vi "Image_Pro_controls_from_string.vi"(11 "Setup String":string) -> (0 "ROI to crop (pixels)":T2={"Xmax"=2147483647, "Ymax"=2147483647, "Xmin"=0, "Ymin"=0}, 1 "Txy range (pixels)":T3={"Tx max (pix)"=2147483647, "Tx min (pix)"=-2147483648, "Ty max (pix)"=2147483647, "Ty min (pix)"=-2147483648}, 2 "Theta range (deg)":T5={"theta max (deg)"=180.0, "theta min (deg)"=-180.0} {"theta min (deg)" min=-360.0 max=360.0; "theta max (deg)" min=-360.0 max=360.0}, 3 "Controls":T4={"Auto ROI (for rot.)"=FALSE, "Apply scaling"=FALSE, "Apply rotation"=TRUE, "Apply Tx"=TRUE, "Apply Ty"=TRUE, "Keep proc. img"=FALSE}, 4 "Camera":string, 5 "Quality":u32=750 max=1000, 7 "Resolution":T1 items=["Low", "Med.", "High", "Max."])   [LabVIEW 2015]
uses:
  Typedefs/Theta range.ctl
  Typedefs/Top level controls.ctl
  Typedefs/Txy range.ctl
  Typedefs/ROI bounds.ctl
  Camera Server/Camera enum/Camera resolution.ctl
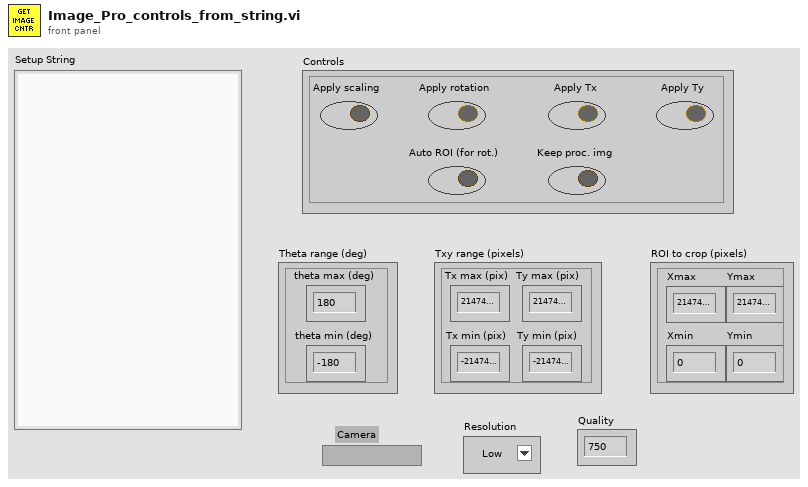
[diagram p1: front panel]
types:
  T1 = typedef "Camera resolution.ctl" = u8
  T2 = typedef "ROI bounds.ctl" = cluster{"Xmax":i32, "Ymax":i32, "Xmin":i32, "Ymin":i32}
  T3 = typedef "Txy range.ctl" = cluster{"Tx max (pix)":i32, "Tx min (pix)":i32, "Ty max (pix)":i32, "Ty min (pix)":i32}
  T4 = typedef "Top level controls.ctl" = cluster{"Auto ROI (for rot.)":bool, "Apply scaling":bool, "Apply rotation":bool, "Apply Tx":bool, "Apply Ty":bool, "Keep proc. img":bool}
  T5 = typedef "Theta range.ctl" = cluster{"theta max (deg)":dbl, "theta min (deg)":dbl}
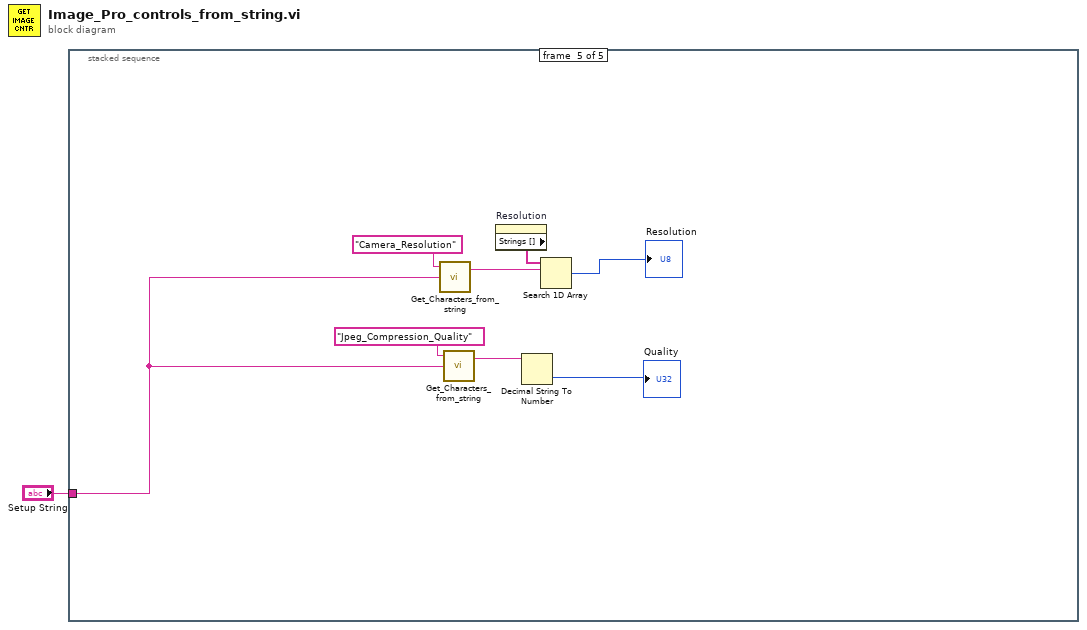
[diagram p0: block diagram]
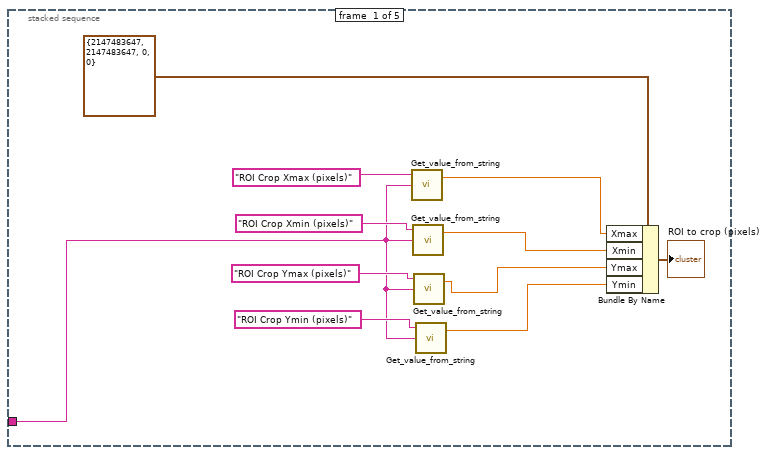
[diagram p2: hidden frame]
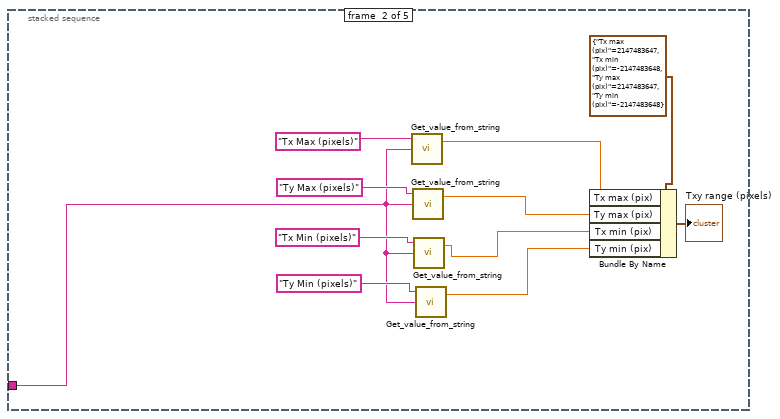
[diagram p3: hidden frame]
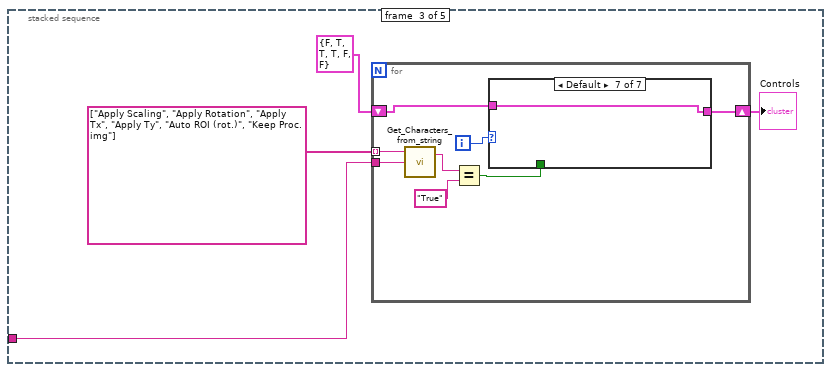
[diagram p4: hidden frame]
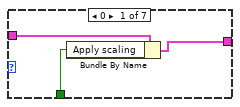
[diagram p5: hidden frame]
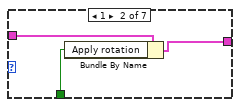
[diagram p6: hidden frame]
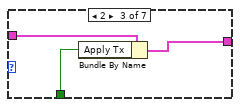
[diagram p7: hidden frame]
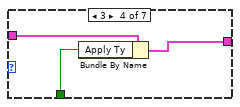
[diagram p8: hidden frame]
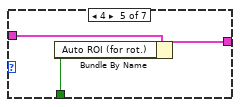
[diagram p9: hidden frame]
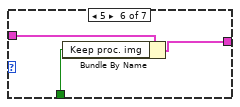
[diagram p10: hidden frame]
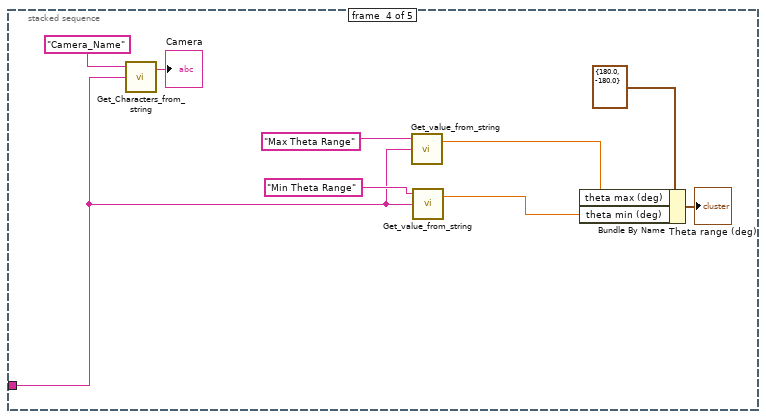
[diagram p11: hidden frame]
diagram:
  n1 = stacked-sequence {
    tunnel: "Setup String" -> [w2 w13 w24 w55 w69]
    frame #0 {
      n2 = call "Get_value_from_string.vi"("Input string"=w2, "Variable name"="ROI Crop Xmax (pixels)" ("Label for characters")) -> ("Value"=w7:dbl)  [unwired: 1 in, 1 out]
      n3 = call "Get_value_from_string.vi"("Input string"=w2, "Variable name"="ROI Crop Xmin (pixels)" ("Label for characters")) -> ("Value"=w6:dbl)  [unwired: 1 in, 1 out]
      n4 = call "Get_value_from_string.vi"("Input string"=w2, "Variable name"="ROI Crop Ymax (pixels)" ("Label for characters")) -> ("Value"=w5:dbl)  [unwired: 1 in, 1 out]
      n5 = call "Get_value_from_string.vi"("Input string"=w2, "Variable name"="ROI Crop Ymin (pixels)" ("Label for characters")) -> ("Value"=w4:dbl)  [unwired: 1 in, 1 out]
      n6 = Bundle By Name(cluster=T2 {"Xmax"=2147483647, "Ymax"=2147483647, "Xmin"=0, "Ymin"=0} ("ROI to crop (pixels)"), "Xmax"=w7, "Xmin"=w6, "Ymax"=w5, "Ymin"=w4) -> (→"ROI to crop (pixels)":T2)
    }
    frame #1 {
      n7 = call "Get_value_from_string.vi"("Input string"=w13, "Variable name"="Tx Max (pixels)" ("Label for characters")) -> ("Value"=w19:dbl)  [unwired: 1 in, 1 out]
      n8 = call "Get_value_from_string.vi"("Input string"=w13, "Variable name"="Ty Max (pixels)" ("Label for characters")) -> ("Value"=w18:dbl)  [unwired: 1 in, 1 out]
      n9 = call "Get_value_from_string.vi"("Input string"=w13, "Variable name"="Tx Min (pixels)" ("Label for characters")) -> ("Value"=w17:dbl)  [unwired: 1 in, 1 out]
      n10 = call "Get_value_from_string.vi"("Input string"=w13, "Variable name"="Ty Min (pixels)" ("Label for characters")) -> ("Value"=w16:dbl)  [unwired: 1 in, 1 out]
      n11 = Bundle By Name(cluster=T3 {"Tx max (pix)"=2147483647, "Tx min (pix)"=-2147483648, "Ty max (pix)"=2147483647, "Ty min (pix)"=-2147483648} ("Txy range (pixels)"), "Tx max (pix)"=w19, "Ty max (pix)"=w18, "Tx min (pix)"=w17, "Ty min (pix)"=w16) -> (→"Txy range (pixels)":T3)
    }
    frame #2 {
      n12 = for {
        tunnel: string[] ["Apply Scaling", "Apply Rotation", "Apply Tx", "Apply Ty", "Auto ROI (rot.)", "Keep Proc. img"] -> [w35] mode=indexing
        tunnel: w24 -> [w34]
        shift-right: [w32] -> w25
        shift-left: T4 {"Auto ROI (for rot.)"=FALSE, "Apply scaling"=TRUE, "Apply rotation"=TRUE, "Apply Tx"=TRUE, "Apply Ty"=FALSE, "Keep proc. img"=FALSE} ("Controls") -> [w33]
        i -> [w29]
        n13 = call "Get_Characters_from_string.vi"("Input string"=w34, "Variable name"=w35) -> ("Value"=w31:string)  [unwired: 1 in, 1 out]
        n14 = Equal?(x=w31, y="True") -> (x = y?=w28:bool)
        n15 = case shown="Default" w29 {
          tunnel: w33 -> [w38 w41 w44 w47 w50 w53 w54]
          tunnel: [w37 w40 w43 w46 w49 w52 w54] -> w32
          tunnel: w28 -> [w36 w39 w42 w45 w48 w51 _]
          frame 0 {
            n16 = Bundle By Name(cluster=w38, "Apply scaling"=w36) -> (w37:T4)
          }
          frame 1 {
            n17 = Bundle By Name(cluster=w41, "Apply rotation"=w39) -> (w40:T4)
          }
          frame 2 {
            n18 = Bundle By Name(cluster=w44, "Apply Tx"=w42) -> (w43:T4)
          }
          frame 3 {
            n19 = Bundle By Name(cluster=w47, "Apply Ty"=w45) -> (w46:T4)
          }
          frame 4 {
            n20 = Bundle By Name(cluster=w50, "Auto ROI (for rot.)"=w48) -> (w49:T4)
          }
          frame 5 {
            n21 = Bundle By Name(cluster=w53, "Keep proc. img"=w51) -> (w52:T4)
          }
          frame Default {
          }
        }
      }
      "Controls" <- w25
    }
    frame #3 {
      n22 = call "Get_Characters_from_string.vi"("Input string"=w55, "Variable name"="Camera_Name" ("Label for characters")) -> ("Value"=→"Camera":string)  [unwired: 1 in, 1 out]
      n23 = call "Get_value_from_string.vi"("Input string"=w55, "Variable name"="Max Theta Range" ("Label for characters")) -> ("Value"=w60:dbl)  [unwired: 1 in, 1 out]
      n24 = call "Get_value_from_string.vi"("Input string"=w55, "Variable name"="Min Theta Range" ("Label for characters")) -> ("Value"=w59:dbl)  [unwired: 1 in, 1 out]
      n25 = Bundle By Name(cluster=T5 {"theta max (deg)"=180.0, "theta min (deg)"=-180.0} ("Theta range (deg)"), "theta max (deg)"=w60, "theta min (deg)"=w59) -> (→"Theta range (deg)":T5)
    }
    frame #4 {
      n26 = call "Get_Characters_from_string.vi"("Input string"=w69, "Variable name"="Camera_Resolution" ("Label for characters")) -> ("Value"=w65:string)  [unwired: 1 in, 1 out]
      n27 = call "Get_Characters_from_string.vi"("Input string"=w69, "Variable name"="Jpeg_Compression_Quality" ("Label for characters")) -> ("Value"=w68:string)  [unwired: 1 in, 1 out]
      n28 = property on="Resolution" class="Ring (strict)"() -> ("Strings []"=w66:string[])  [unwired: 2 in, 2 out]
      n29 = Decimal String To Number(string=w68) -> (number=→"Quality":i32)  [unwired: 2 in, 1 out]
      n30 = Search 1D Array(1D array=w66, element=w65) -> (index of element=→"Resolution":i32)  [unwired: 1 in]
    }
  }
